vi "SortDAQchassisWithIP.vi"(8 "error in (no error)":errorcluster, 11 "Target (localhost)":refnum<k21>="localhost") -> (0 "error out":errorcluster, 2 "SN Number":string[](array[string]))   [LabVIEW 2017, in "TSNcDAQ_AI.lvlib"]
uses:
  <vilib>/addons/InsightCM/Devices/Shared/Cms/DAQmx/TSNcDAQ_AI.lvlib
  <vilib>/nisyscfg/Close (System).vi
  <resource>/objmgr/nicontrollersysapi.rc
  <vilib>/nisyscfg/nisyscfg.lvlib
  <resource>/objmgr/niflexrioatomicsae.rc
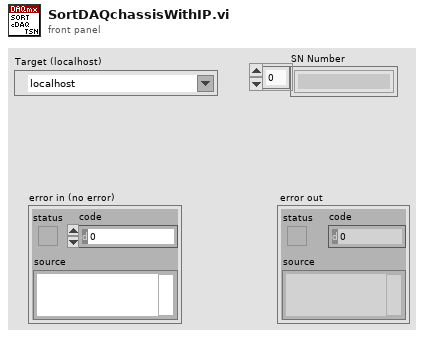
[diagram p1: front panel]
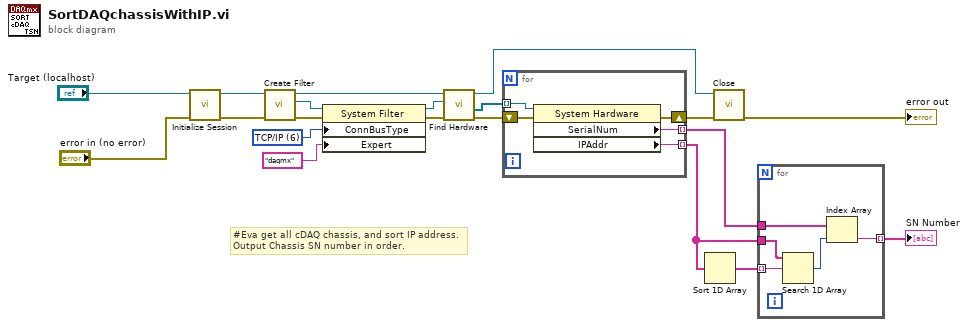
[diagram p0: block diagram]
diagram:
  w14 = u32 6 items=["BuiltIn/System", "PXI/PCI", "USB", "GPIB", "VXI", "Serial", "TCP/IP", "cRIO", "SCXI", "cDAQ", "SwitchBlock", "SCC", "FireWire", "Accessory", "CAN", "SwitchBlock Device"] ("Devices & Chassis:Connects To Bus Type")
  # "#Eva get all cDAQ chassis, and sort IP address.\nOutput Chassis SN number in order."
  n1 = call <vilib>:"Initialize Session.vi"("error in (no error)"="error in (no error)", "Target (localhost)"="Target (localhost)") -> ("error out"=w3:errorcluster, "Session out"=w7:refnum<k21>)  [unwired: 8 in]
  n2 = call <vilib>:"Create Filter.vi"("error in (no error)"=w3, "Session in"=w7) -> ("error out"=w19:errorcluster, "Filter out"=w11:refnum<k20>, "Session out"=w12:refnum<k21>)  [unwired: 7 in]
  n3 = property class="System Filter"(reference=w11, error in=w19, "ConnBusType"=w14, "Expert"="daqmx" ("Expert Info:Expert Name")) -> (reference out=w13:refnum<k20>, error out=w20:errorcluster)
  n4 = call <vilib>:"Find Hardware.vi"("error in (no error)"=w20, "Filter in"=w13, "Session in"=w12) -> ("error out"=w9:errorcluster, "Resources out"=w10:refnum<k20>[], "Session out"=w5:refnum<k21>)  [unwired: 1 in, 5 out]
  n5 = for {
    tunnel: w10 -> [w25] mode=indexing
    shift-right: [w23] -> w4
    shift-left: w9 -> [w24]
    tunnel: [w22] -> w18 mode=indexing
    tunnel: [w21] -> w17 mode=indexing
    n6 = property class="System Hardware"(reference=w25, error in=w24) -> (error out=w23:errorcluster, "SerialNum"=w22:string, "IPAddr"=w21:string)  [unwired: 1 out]
  }
  n7 = Sort 1D Array(array=w17) -> (sorted array=w16:string[])
  n8 = call-poly <vilib>:"Close.vi"("error in (no error)"=w4, "Session in"=w5) -> ("error out"=→"error out":errorcluster)  [unwired: 9 in]
  n9 = for {
    tunnel: w16 -> [w29] mode=indexing
    tunnel: w17 -> [w30]
    tunnel: w18 -> [w28]
    tunnel: [w26] -> w6 mode=indexing
    n10 = Search 1D Array(1D array=w30, element=w29) -> (index of element=w27:i32)  [unwired: 1 in]
    n11 = Index Array(array=w28, index=w27) -> (element=w26:string)
  }
  "SN Number" <- w6
